vi "4_3.vi"() -> ()   [LabVIEW 2020]
uses:
  <vilib>/numeric/Random Number (Range) DBL.vi
panel:
  out "Average":dbl
  out "output array":dbl[][](array[numeric])
  in  "OK Button":bool
  in  "Set value":dbl
  in  "Column":i32
  in  "Row":i32
  out "subarray":dbl[][](array[numeric])
  out "Array":dbl[][](array[numeric])
  in  "Num of columns":i32
  in  "Num of rows":i32
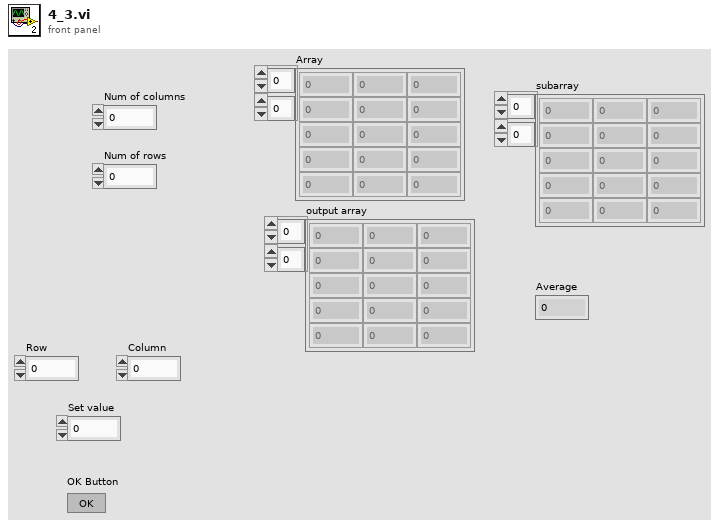
[diagram p1: front panel]
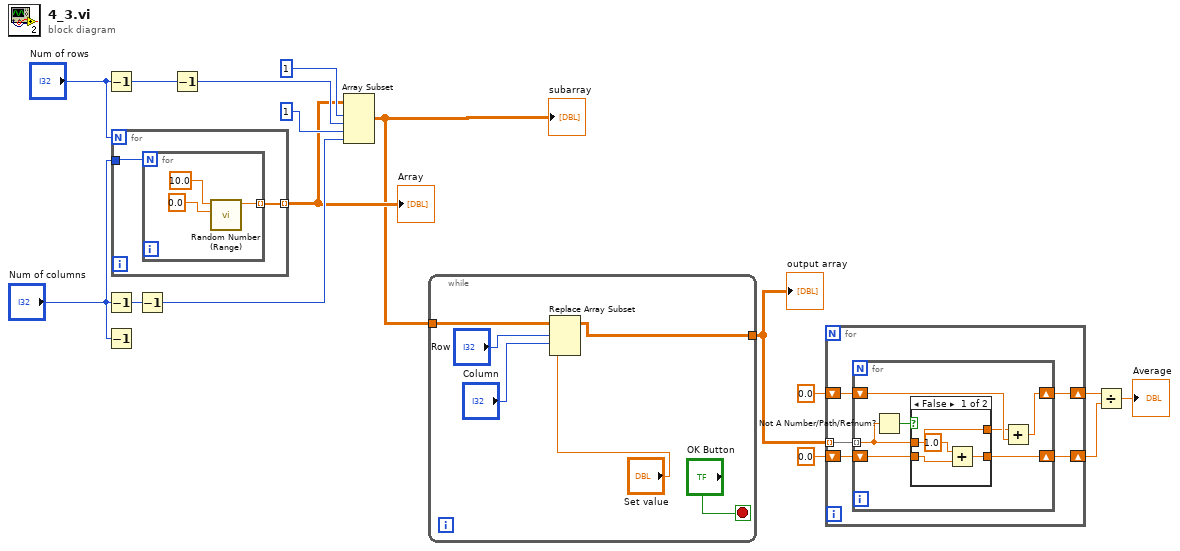
[diagram p0: block diagram]
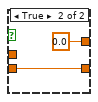
[diagram p2: hidden frame]
diagram:
  n1 = Decrement(x="Num of rows") -> (x-1=w9:i32)
  n2 = Decrement(x="Num of columns") -> (x-1=w10:i32)
  n3 = Decrement(x="Num of columns") -> ()  [unwired: 1 out]
  n4 = for {
    N: "Num of rows" -> [_]
    tunnel: "Num of columns" -> [w18]
    tunnel: [w17] -> w8 mode=indexing
    n5 = for {
      N: w18 -> [_]
      tunnel: [w19] -> w17 mode=indexing
      n6 = call-poly <vilib>:"Random Number (Range).vi"("lower bound (0)"=0.0, "upper bound (100)"=10.0) -> ("number"=w19:dbl)  [unwired: 9 in]
    }
  }
  "Array" <- w8
  n7 = Decrement(x=w10) -> (x-1=w11:i32)
  n8 = Decrement(x=w9) -> (x-1=w14:i32)
  n9 = Array Subset(array=w8, index (row)=1 ("index"), length (row)=w14, index (col)=1 ("index"), length (col)=w11) -> (w7:dbl[][])
  "subarray" <- w7
  n10 = while {
    tunnel: w7 -> [w27]
    tunnel: [w22] -> w5
    stop <- "OK Button" stop-if-true
    n11 = Replace Array Subset(array=w27, new element="Set value", index (row)="Row", index (col)="Column") -> (w22:dbl[][])
  }
  "output array" <- w5
  n12 = for {
    shift-right: [w31] -> w2
    shift-left: 0.0 -> [w30]
    tunnel: w5 -> [w32] mode=indexing
    shift-right: [w29] -> w1
    shift-left: 0.0 -> [w28]
    n13 = for {
      shift-right: [w39] -> w31
      shift-left: w30 -> [w38]
      tunnel: w32 -> [w33] mode=indexing
      shift-right: [w36] -> w29
      shift-left: w28 -> [w35]
      n14 = Not A Number/Path/Refnum?(number/path/refnum=w33) -> (NaN/Path/Refnum?=w34:bool)
      n15 = case shown="False" w34 {
        tunnel: [w43 0.0 ("number")] -> w37
        tunnel: w33 -> [w43 _]
        tunnel: [w42 w44] -> w36
        tunnel: w35 -> [w41 w44]
        frame False {
          n16 = Add(x=1.0, y=w41) -> (x+y=w42:dbl)
        }
        frame True {
        }
      }
      n17 = Add(x=w37, y=w38) -> (x+y=w39:dbl)
    }
  }
  n18 = Divide(x=w2, y=w1) -> (x/y=→"Average":dbl)
